vi "attempt scanivalve connection.vi"(7 "RT Queues":T8, 11 "Comms data in":T1={"Parameters"={"error writer name"="", "command reader name"="", "error buffer size"=0, "command buffer size"=0, "scanivalveIP"="", "scanivalvePeriod"=16}, "Variables"={"listen schedule"=0, "incident buffer"=[], "command stream"="", "error stream"="", "waiting for command stream connect"=FALSE, "waiting for error stream connect"=FALSE, "scanivalve connection"=refnum, "scanivalveScheduleID"=16, "activeScanivalvePorts"=[], "channelCount"=0}, "scanivalveConfig"={"listS"={"period"=0, "ADtrig"=FALSE, "ScanTrig"=FALSE, "page"=0, "qpkts"=0}, "listC"={"ZC"=FALSE, "unitScan"="", "CvtUnit"=0.0, "bin"=FALSE, "EU"=FALSE}, "listSG"={"Avg1"=0, "FPS1"=0, "SGEnable1"=FALSE}, "activeChannels"={"Chan1"={"101"=FALSE, "102"=FALSE, "103"=FALSE, "104"=FALSE, "109"=FALSE, "110"=FALSE, "111"=FALSE, "112"=FALSE, "201"=FALSE, "202"=FALSE, "203"=FALSE, "204"=FALSE, "209"=FALSE, "210"=FALSE, "211"=FALSE, "212"=FALSE, "301"=FALSE, "302"=FALSE, "303"=FALSE, "304"=FALSE, "309"=FALSE, "310"=FALSE, "311"=FALSE, "312"=FALSE, "401"=FALSE, "402"=FALSE, "403"=FALSE, "404"=FALSE, "409"=FALSE, "410"=FALSE, "411"=FALSE, "412"=FALSE}}}}) -> (3 "Comms data out":T1={"Parameters"={"error writer name"="", "command reader name"="", "error buffer size"=0, "command buffer size"=0, "scanivalveIP"="", "scanivalvePeriod"=16}, "Variables"={"listen schedule"=0, "incident buffer"=[], "command stream"="", "error stream"="", "waiting for command stream connect"=FALSE, "waiting for error stream connect"=FALSE, "scanivalve connection"=refnum, "scanivalveScheduleID"=16, "activeScanivalvePorts"=[], "channelCount"=0}, "scanivalveConfig"={"listS"={"period"=0, "ADtrig"=FALSE, "ScanTrig"=FALSE, "page"=0, "qpkts"=0}, "listC"={"ZC"=FALSE, "unitScan"="", "CvtUnit"=0.0, "bin"=FALSE, "EU"=FALSE}, "listSG"={"Avg1"=0, "FPS1"=0, "SGEnable1"=FALSE}, "activeChannels"={"Chan1"={"101"=FALSE, "102"=FALSE, "103"=FALSE, "104"=FALSE, "109"=FALSE, "110"=FALSE, "111"=FALSE, "112"=FALSE, "201"=FALSE, "202"=FALSE, "203"=FALSE, "204"=FALSE, "209"=FALSE, "210"=FALSE, "211"=FALSE, "212"=FALSE, "301"=FALSE, "302"=FALSE, "303"=FALSE, "304"=FALSE, "309"=FALSE, "310"=FALSE, "311"=FALSE, "312"=FALSE, "401"=FALSE, "402"=FALSE, "403"=FALSE, "404"=FALSE, "409"=FALSE, "410"=FALSE, "411"=FALSE, "412"=FALSE}}}})   [LabVIEW 2018]
uses:
  Type Defs/Queues cluster.ctl
  ICL-LabVIEW_General/Message Scheduler/message scheduler.lvclass
  comms data.ctl
  Type Defs/generic incident.ctl
  ICL-LabVIEW_General/Scanivalve API project/full interface/polymorphic/scanivalveConfig.ctl
  ICL-LabVIEW_General/Scanivalve API project/full interface/listS.ctl
  ICL-LabVIEW_General/Scanivalve API project/full interface/listC.ctl
  ICL-LabVIEW_General/Scanivalve API project/full interface/listSG.ctl
  ICL-LabVIEW_General/Scanivalve API project/full interface/chan1.ctl
  ICL-LabVIEW_General/Message Scheduler/generic message queue/standard message queue/standard message.lvclass
  C:/GitHub/ICL-LabVIEW_General/Message Scheduler/generic message queue/generic message.lvclass
  ICL-LabVIEW_General/Scanivalve API project/full interface/polymorphic/connect.vi
  ICL-LabVIEW_General/Scanivalve API project/full interface/polymorphic/check configuration.vi
  ICL-LabVIEW_General/Scanivalve API project/full interface/polymorphic/set channels.vi
  ICL-LabVIEW_General/Scanivalve API project/full interface/polymorphic/start.vi
  Queue VIs/En-queue RT comms element.vi
  ICL-LabVIEW_General/Message Scheduler/scheduled message/scheduled message.lvclass
  ICL-LabVIEW_General/Scanivalve API project/Scanivalve API.lvlib
types:
  T1 = typedef "comms data.ctl" = cluster{"Parameters":cluster{"error writer name":string, "command reader name":string, "error buffer size":i32, "command buffer size":i32, "scanivalveIP":string, "scanivalvePeriod":u16}, "Variables":cluster{"listen schedule":u32, "incident buffer":T2[], "command stream":refnum<k21>, "error stream":refnum<k21>, "waiting for command stream connect":bool, "waiting for error stream connect":bool, "scanivalve connection":refnum<k5>, "scanivalveScheduleID":u32, "activeScanivalvePorts":i32[], "channelCount":i16}, "scanivalveConfig":T3}
  T2 = typedef "generic incident.ctl" = cluster{"timestamp":timestamp, "type":string, "Variant":variant}
  T3 = typedef "Scanivalve API.lvlib/scanivalveConfig.ctl" = cluster{"listS":T4, "listC":T5, "listSG":T6, "activeChannels":T7}
  T4 = typedef "Scanivalve API.lvlib/listS.ctl" = cluster{"period":u16, "ADtrig":bool, "ScanTrig":bool, "page":u16, "qpkts":u16}
  T5 = typedef "Scanivalve API.lvlib/listC.ctl" = cluster{"ZC":bool, "unitScan":string, "CvtUnit":dbl, "bin":bool, "EU":bool}
  T6 = typedef "Scanivalve API.lvlib/listSG.ctl" = cluster{"Avg1":u16, "FPS1":u16, "SGEnable1":bool}
  T7 = typedef "Scanivalve API.lvlib/chan1.ctl" = cluster{"Chan1":cluster{"101":bool, "102":bool, "103":bool, "104":bool, "109":bool, "110":bool, "111":bool, "112":bool, "201":bool, "202":bool, "203":bool, "204":bool, "209":bool, "210":bool, "211":bool, "212":bool, "301":bool, "302":bool, "303":bool, "304":bool, "309":bool, "310":bool, "311":bool, "312":bool, "401":bool, "402":bool, "403":bool, "404":bool, "409":bool, "410":bool, "411":bool, "412":bool}}
  T8 = typedef "Queues cluster.ctl" = cluster{"RT Message":refnum<queue>, "RT Comms":refnum<queue>, "RT Data":refnum<queue>, "RT FIFO":refnum<queue>, "message scheduler":refnum<class "message scheduler.lvclass">}
  T9 = enum16{"ASCII on demand", "binary on demand", "binary high-speed"}
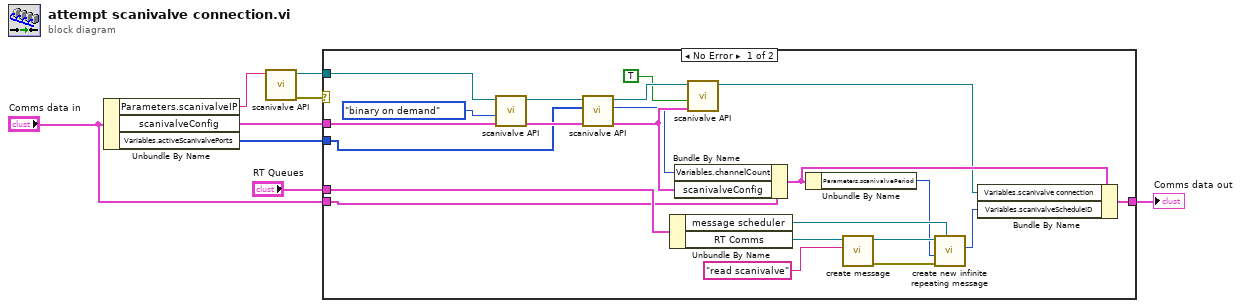
[diagram p0: block diagram]
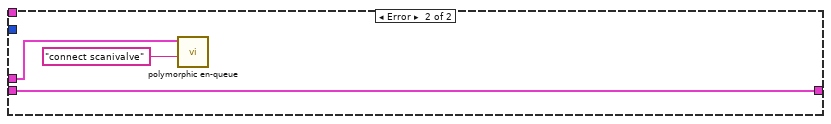
[diagram p2: hidden frame]
diagram:
  n1 = Unbundle By Name("Comms data in") -> ("Parameters.scanivalveIP"=w6:string, "scanivalveConfig"=w2:T3, "Variables.activeScanivalvePorts"=w3:i32[])
  n2 = call-poly "scanivalve API.vi"("address"=w6) -> ("error out 2"=w5:errorcluster, "connection ID"=w1:refnum<k5>)  [unwired: 9 in]
  n3 = case shown="No Error" w5 {
    tunnel: [w30 w31] -> w7
    tunnel: "RT Queues" -> [w29 w33]
    tunnel: "Comms data in" -> [w17 w31]
    tunnel: w3 -> [w15 _]
    tunnel: w2 -> [w14 _]
    tunnel: w1 -> [w13 _]
    frame No Error {
      n4 = call-poly "scanivalve API.vi"("scanivalveConfig"=w14, "config"=T9."binary on demand", "connection in"=w13) -> ("output cluster"=w18:T3, "connection out"=w19:refnum<k5>)  [unwired: 6 in, 1 out]
      n5 = call-poly "scanivalve API.vi"("scanivalveConfig"=w18, "activeChannels"=w15, "connection in"=w19) -> ("scanivalveConfig"=w21:T3, "channelCount"=w9:i16, "connection out"=w20:refnum<k5>)  [unwired: 6 in]
      n6 = Unbundle By Name(w29) -> ("message scheduler"=w28:refnum<class "message scheduler.lvclass">, "RT Comms"=w27:refnum<queue>)
      n7 = Bundle By Name(cluster=w17, "Variables.channelCount"=w9, "scanivalveConfig"=w21) -> (w12:T1)
      n8 = call-poly "scanivalve API.vi"("scanivalveConfig"=w21, "Scan"=TRUE, "connection in"=w20) -> ("connection out"=w11:refnum<k5>)  [unwired: 8 in]
      n9 = Unbundle By Name(w12) -> ("Parameters.scanivalvePeriod"=w24:u16)
      n10 = call "create message.vi"("message"="read scanivalve", "queue ref"=w27) -> ("error out"=w23:errorcluster, "standard message out"=w26:refnum<class "standard message.lvclass">)  [unwired: 8 in]
      n11 = call "create new infinite repeating message.vi"("message scheduler"=w28, "error in (no error)"=w23, "ms delay"=w24, "message"=w26) -> ("schedule ID"=w22:u32)  [unwired: 6 in, 1 out]
      n12 = Bundle By Name(cluster=w12, "Variables.scanivalve connection"=w11, "Variables.scanivalveScheduleID"=w22) -> (w30:T1)
    }
    frame Error {
      n13 = call-poly "polymorphic en-queue.vi"("Message"="connect scanivalve", "RT Queues"=w33) -> ()  [unwired: 9 in, 1 out]
    }
  }
  "Comms data out" <- w7
